vi "TextToLines.vi"(8 "error in (no error)":errorcluster, 11 "string":string) -> (0 "error out":errorcluster, 3 "Lines":string[](array[string]))   [LabVIEW 2012]
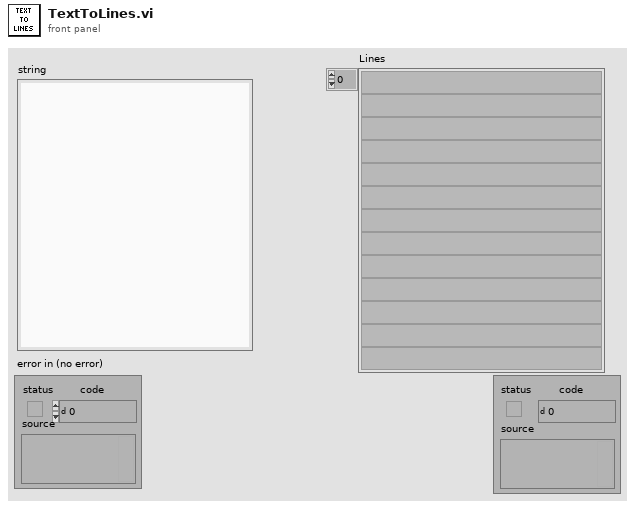
[diagram p1: front panel]
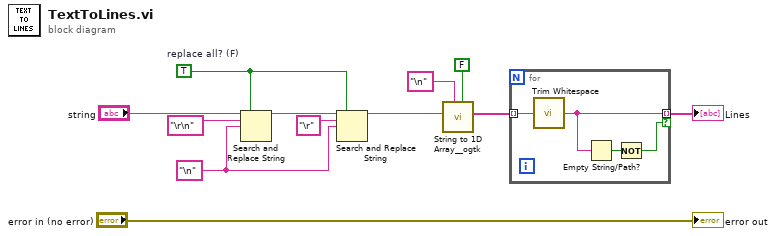
[diagram p0: block diagram]
diagram:
  w3 = TRUE  # replace all? (F)
  w4 = "\n" ("delimiter (Tab)")
  n1 = Search and Replace String(replace all?=w3, input string="string", search string="\r\n" ("delimiter (Tab)"), replace string=w4) -> (result string=w7:string)  [unwired: 4 in, 3 out]
  n2 = Search and Replace String(replace all?=w3, input string=w7, search string="\r" ("delimiter (Tab)"), replace string=w4) -> (result string=w5:string)  [unwired: 4 in, 3 out]
  n3 = call <userlib>:"String to 1D Array__ogtk.vi"("ignore duplicate delimiters? (F=No)"=FALSE, "delimiter (Tab)"="\n", "string"=w5) -> ("Array of Strings"=w8:string[])  [unwired: 8 in]
  n4 = for {
    tunnel: w8 -> [w16] mode=indexing
    tunnel: [w15] -> w11 mode=indexing if=w13
    n5 = call <vilib>:"Trim Whitespace.vi"("string"=w16) -> ("trimmed string"=w15:string)  [unwired: 1 in]
    n6 = Empty String/Path?(string/path=w15) -> (empty?=w14:bool)
    n7 = Not(x=w14) -> (.not. x?=w13:bool)
  }
  "Lines" <- w11
  "error out" <- "error in (no error)"
